vi "set Message Channel.vi"(10 "Message Channel":refnum<user-event>, 11 "Actor API in":refnum<class "Actor API.lvclass">) -> (3 "Actor API out":refnum<class "Actor API.lvclass">)   [LabVIEW 2020, in "Actor API.lvclass"]
uses:
  Actor API.lvclass
  Actor/Message.ctl
  Actor API.lvclass/Actor API.ctl
  Actor/Actor.lvclass
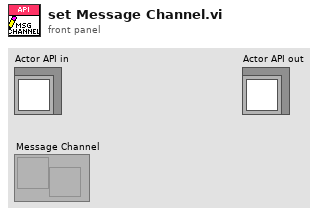
[diagram p1: front panel]
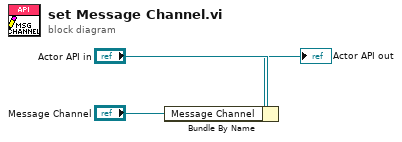
[diagram p0: block diagram]
diagram:
  n1 = Bundle By Name(cluster="Actor API in", "Message Channel"="Message Channel") -> (→"Actor API out":refnum<class "Actor API.lvclass">)
